vi "Part 2.vi"() -> ()   [LabVIEW 2021]
panel:
  in  "Input":string
  out "Output":i64
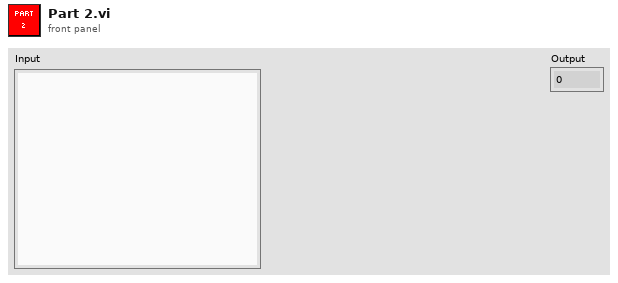
[diagram p1: front panel]
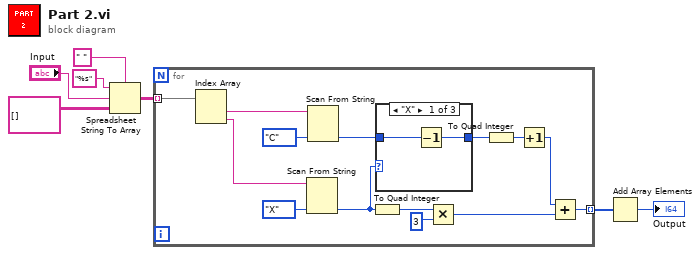
[diagram p0: block diagram]
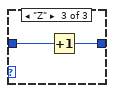
[diagram p3: hidden frame]
diagram:
  n1 = Spreadsheet String To Array(delimiter (Tab)=" ", format string="%s", spreadsheet string="Input", array type (2D Dbl)=string[][] []) -> (array=w3:string[][])
  n2 = for {
    tunnel: w3 -> [w21] mode=indexing
    tunnel: [w16] -> w2 mode=indexing
    n3 = Index Array(array=w21) -> (element #1=w18:string, element #2=w20:string)  [unwired: 2 in]
    n4 = Scan From String(input string=w20, default 1=enum16{"X", "Y", "Z"}."X") -> (output 1=w15:enum16{"X", "Y", "Z"})  [unwired: 3 in, 3 out]
    n5 = Scan From String(input string=w18, default 1=enum16{"A", "B", "C"}."C") -> (output 1=w17:enum16{"A", "B", "C"})  [unwired: 3 in, 3 out]
    n6 = To Quad Integer(1:w15) -> (0:w10:i64)
    n7 = case shown="\"X\"" w15 {
      tunnel: w17 -> [w23 w24 w26]
      tunnel: [w22 w24 w25] -> w13
      frame "X" {
        n8 = Decrement(x=w23) -> (x-1=w22:enum16{"A", "B", "C"})
      }
      frame "Y" {
      }
      frame "Z" {
        n9 = Increment(x=w26) -> (x+1=w25:enum16{"A", "B", "C"})
      }
    }
    n10 = Multiply(x=w10, y=i64 3) -> (x*y=w9:i64)
    n11 = To Quad Integer(1:w13) -> (0:w12:i64)
    n12 = Increment(x=w12) -> (x+1=w11:i64)
    n13 = Add(x=w11, y=w9) -> (x+y=w16:i64)
  }
  n14 = Add Array Elements(numeric array=w2) -> (sum=→"Output":i64)
